vi "Untitled 4.vi"() -> ()   [LabVIEW 2017, in "labview-standard-library.lvlib" / "file-transfer.lvlib"]
uses:
  file-transfer.lvlib
  <vilib>/FTP/NI_FTP.lvlib
panel:
  out "error out":errorcluster
  out "file errors":errorcluster[](array[cluster])
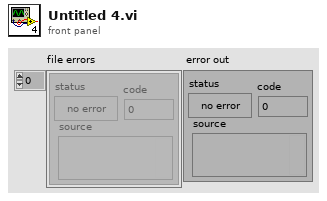
[diagram p1: front panel]
types:
  T1 = cluster{"remote path":string, "local path":path, "binary":bool}[]
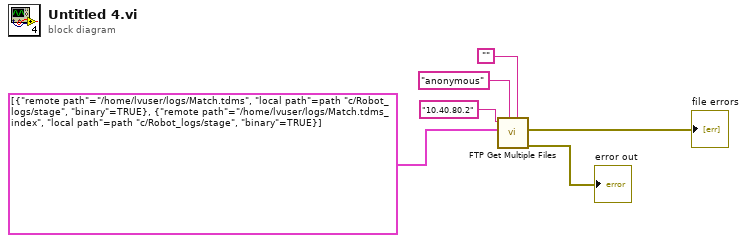
[diagram p0: block diagram]
diagram:
  n1 = call <vilib>:"FTP Get Multiple Files.vi"("password"="", "user"="anonymous", "file specifications"=T1 [{"remote path"="/home/lvuser/logs/Match.tdms", "local path"=path "c:/Robot_logs/stage", "binary"=TRUE}, {"remote path"="/home/lvuser/logs/Match.tdms_index", "local path"=path "c:/Robot_logs/stage", "binary"=TRUE}], "host"="10.40.80.2") -> ("error out"=→"error out":errorcluster, "file errors"=→"file errors":errorcluster[])  [unwired: 6 in]
